vi "CallbackOnLoadUI.vi"(8 "error in":errorcluster, 11 "node":refnum<data-value>) -> (0 "error out":errorcluster)   [LabVIEW 2023, in "CEF.lvlib" / "CEF_Node.lvclass"]
doc: "Copyright 2017 National Instruments Corporation\n\nLicensed under the Apache License, Version 2.0 (the \"License\"); you may not use this file except in compliance with the License. You may obtain a copy of the License at http://www.apache.org/licenses/LICENSE-2.0\nUnless required by applicable law or agreed to in writing, software distributed under the License is distributed on an \"AS IS\" BASIS, WITHOUT WARRANTIES OR CONDITIONS OF ANY KIND, either express or implied. See the License for the specific language governing permissions and limitations under the License."
uses:
  CEF_Node.lvclass
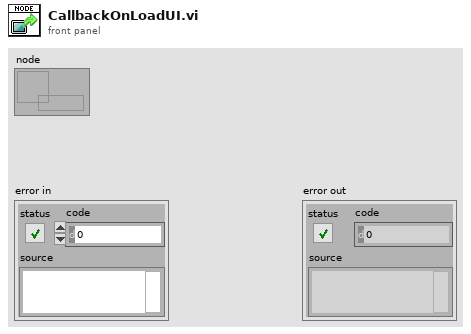
[diagram p1: front panel]
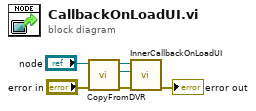
[diagram p0: block diagram]
diagram:
  n1 = call "CopyFromDVR.vi"("error in"="error in", "node in"="node") -> ("error out"=w4:errorcluster, "CEF_Node out"=w2:refnum<class "CEF_Node.lvclass">, "node out"=w1:refnum<data-value>)  [unwired: 7 in]
  n2 = call-dynamic "InnerCallbackOnLoadUI.vi"("error in"=w4, "node (for type)"=w2, "node reference"=w1) -> ("error out"=→"error out":errorcluster)  [unwired: 8 in]
